vi "删除实验.vi"   [LabVIEW 2018]
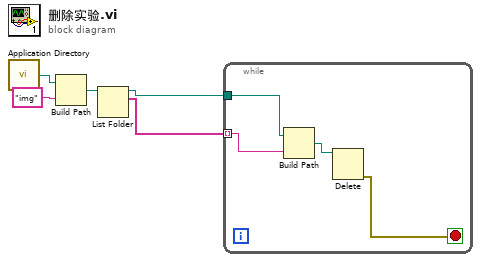
[diagram p0: block diagram]
diagram:
  n1 = call <vilib>:"Application Directory.vi"() -> ("Application Directory"=w5:path)
  n2 = Build Path(base path=w5, name or relative path="img" ("名称或相对路径")) -> (appended path=w3:path)
  n3 = List Folder(path=w3) -> (path out=w2:path, filenames=w1:string[])  [unwired: 3 in, 2 out]
  n4 = while {
    tunnel: w2 -> [w8]
    tunnel: w1 -> [w7] mode=indexing
    stop <- w9 stop-if-true
    n5 = Build Path(base path=w8, name or relative path=w7) -> (appended path=w6:path)
    n6 = Delete(path (use dialog)=w6) -> (error out=w9:errorcluster)  [unwired: 4 in, 2 out]
  }
